vi "Release-message-queues.vi"(8 "error in":errorcluster, 11 "Data ref. in":refnum<data-value>) -> (0 "error IO":errorcluster, 3 "Data ref.":refnum<data-value>)   [LabVIEW 2013, in "CameraVision.lvlib" / "CV-Main.lvclass"]
uses:
  CV-Main.lvclass
  CV-Main.lvclass/CV-Main.ctl
  Read Action queue.vi
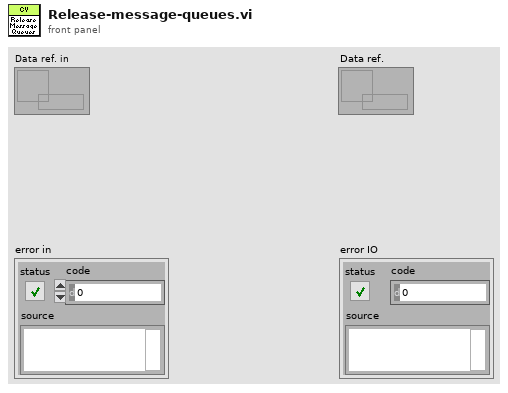
[diagram p1: front panel]
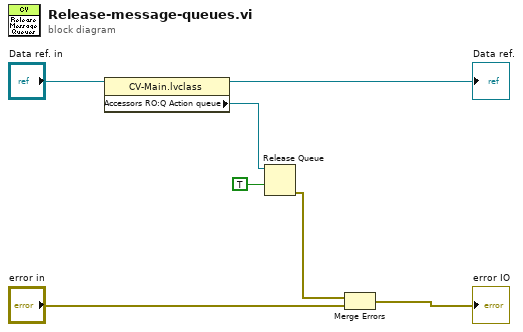
[diagram p0: block diagram]
diagram:
  n1 = property class="CV-Main.lvclass"(reference="Data ref. in") -> (reference out=→"Data ref.":refnum<data-value>, "Accessors RO:Q Action queue"=w2:refnum<queue>)  [unwired: 1 in, 1 out]
  n2 = Release Queue(queue=w2, force destroy? (F)=TRUE) -> (error out=w7:errorcluster)  [unwired: 1 in, 2 out]
  n3 = Merge Errors(w7, "error in") -> (→"error IO":errorcluster)
